vi "gitconfig name.vi"() -> (3 "gitconfig filename":string)   [LabVIEW 2016]
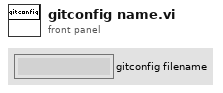
[diagram p1: front panel]
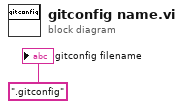
[diagram p0: block diagram]
diagram:
  "gitconfig filename" <- ".gitconfig" ("name or relative path")
